vi "Validate TCP.vi"(8 "error in (no error)":errorcluster, 10 "User TCP Configuration":T1, 11 "LINX Resource":T2={"IO"=enum."Remote", "Interface"=enum."Serial", "LINX Device Config"={"Interface"=enum."Serial", "COM Port"="COM13", "TCP Configuration"={"IP Address"="", "Port"=0}, "Device Family"=1, "Device ID"=1, "Device Name"="myRIO-1900", "TCP Ref"=refnum, "Channels"={"DI"=[0, 1, 2, 3, 4, 5, 6, 7, 8, 9, 10, 11, 12, 13, 14, 15, 16, 17, 18, 19, 20, 21, 22, 23, 24, 25, 26, 27, 28, 29, 30, 31, 32, 33, 34, 35, 36, 37, 38, 39, 40, 41, 42, 43, 44, 45, 46], "DO"=[0, 1, 2, 3, 4, 5, 6, 7, 8, 9, 10, 11, 12, 13, 14, 15, 16, 17, 18, 19, 20, 21, 22, 23, 24, 25, 26, 27, 28, 29, 30, 31, 32, 33, 34, 35, 36, 37, 38, 39, 40, 41, 42, 43, 44, 45, 46], "AI"=[0, 1, 2, 3, 4, 5, 6, 7, 8, 9, 10, 11], "AO"=[], "PWM"=[3, 5, 6, 9, 10], "QE"=[], "UART"=[0, 1], "I2C 2"=[0], "SPI"=[0], "CAN"=[], "Servo"=[], "AI Ref (V)"=0.0, "AI Resolution (Bits)"=0, "AO Ref (V)"=0.0, "AO Resolution (Bits)"=0}}}) -> (0 "error out":errorcluster, 1 "WiFi status":u8, 2 "Board TCP Configuration":T1, 3 "LINX Resource Out":T2={"IO"=enum."Remote", "Interface"=enum."Serial", "LINX Device Config"={"Interface"=enum."Serial", "COM Port"="COM13", "TCP Configuration"={"IP Address"="", "Port"=0}, "Device Family"=1, "Device ID"=1, "Device Name"="myRIO-1900", "TCP Ref"=refnum, "Channels"={"DI"=[0, 1, 2, 3, 4, 5, 6, 7, 8, 9, 10, 11, 12, 13, 14, 15, 16, 17, 18, 19, 20, 21, 22, 23, 24, 25, 26, 27, 28, 29, 30, 31, 32, 33, 34, 35, 36, 37, 38, 39, 40, 41, 42, 43, 44, 45, 46], "DO"=[0, 1, 2, 3, 4, 5, 6, 7, 8, 9, 10, 11, 12, 13, 14, 15, 16, 17, 18, 19, 20, 21, 22, 23, 24, 25, 26, 27, 28, 29, 30, 31, 32, 33, 34, 35, 36, 37, 38, 39, 40, 41, 42, 43, 44, 45, 46], "AI"=[0, 1, 2, 3, 4, 5, 6, 7, 8, 9, 10, 11], "AO"=[], "PWM"=[3, 5, 6, 9, 10], "QE"=[], "UART"=[0, 1], "I2C 2"=[0], "SPI"=[0], "CAN"=[], "Servo"=[], "AI Ref (V)"=0.0, "AI Resolution (Bits)"=0, "AO Ref (V)"=0.0, "AO Resolution (Bits)"=0}}})   [LabVIEW 2019, in "LINXx.lvlib"]
doc: "Throw warning if IP/port do not match"
uses:
  LINXx.lvlib
  <vilib>/MakerHub/LINX/Private/Device/Type Defs/TCP Config.ctl
  <vilib>/MakerHub/LINX/Private/Type Defs/LINX Ref.ctl
  <vilib>/MakerHub/LINX/Private/Type Defs/Platform.ctl
  <vilib>/MakerHub/LINX/Private/Type Defs/Interface.ctl
  <vilib>/MakerHub/LINX/Private/Device/Type Defs/LINX Device Config.ctl
  <vilib>/MakerHub/LINX/Private/Device/Type Defs/Channels.ctl
  <vilib>/Utility/error.llb/Error Cluster From Error Code.vi
  <vilib>/ErrorRing/Error Ring.xnode
  <vilib>/MakerHub/LINX/Private/Device/Device.lvlib
  <vilib>/MakerHub/LINX/LMH-LINX.lvlib
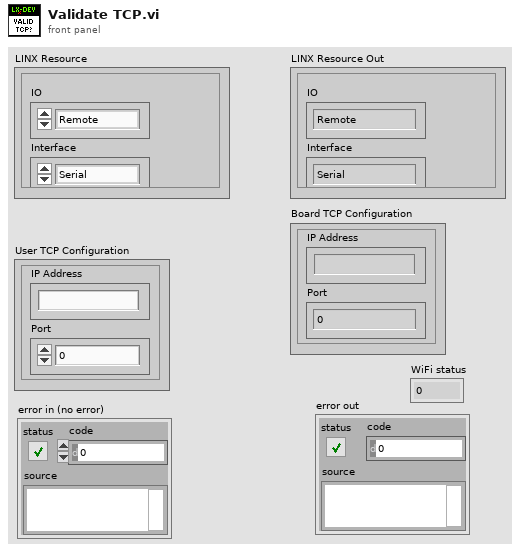
[diagram p1: front panel]
types:
  T1 = typedef "LMH-LINX.lvlib/Device.lvlib/TCP Config.ctl" = cluster{"IP Address":string, "Port":u16}
  T2 = typedef "LMH-LINX.lvlib/LINX Ref.ctl" = cluster{"IO":T3, "Interface":T4, "LINX Device Config":T5}
  T3 = typedef "LMH-LINX.lvlib/Platform.ctl" = enum16{"Remote", "Local"}
  T4 = typedef "LMH-LINX.lvlib/Interface.ctl" = enum16{"Serial", "TCP"}
  T5 = typedef "LMH-LINX.lvlib/Device.lvlib/LINX Device Config.ctl" = cluster{"Interface":T4, "COM Port":refnum<visa-resource-name>, "TCP Configuration":T1, "Device Family":u8, "Device ID":u8, "Device Name":string, "TCP Ref":refnum<k5>, "Channels":T6}
  T6 = typedef "LMH-LINX.lvlib/Channels.ctl" = cluster{"DI":u8[], "DO":u8[], "AI":u8[], "AO":u8[], "PWM":u8[], "QE":u8[], "UART":u8[], "I2C 2":u8[], "SPI":u8[], "CAN":u8[], "Servo":u8[], "AI Ref (V)":dbl, "AI Resolution (Bits)":u8, "AO Ref (V)":dbl, "AO Resolution (Bits)":u8}
  T7 = typedef "LMH-LINX.lvlib/Device.lvlib/Wifi Config.ctl" = cluster{"SSID":string, "IP Address":string, "Port":u16, "WIFI Security Type":T8, "Password":string}
  T8 = typedef "LMH-LINX.lvlib/WIFI Security Type.ctl" = enum8{"None", "WPA2 Password", "WPA2 Key", "WEP40", "WEP104"}
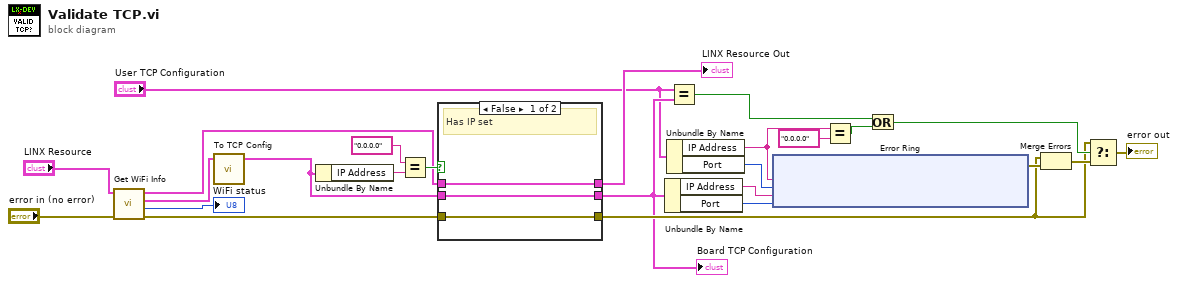
[diagram p0: block diagram]
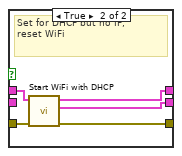
[diagram p2: hidden frame]
diagram:
  n1 = call "Get WiFi Info.vi"("Error In"="error in (no error)", "LINX Resource"="LINX Resource") -> ("Error Out"=w10:errorcluster, "WiFi status"=→"WiFi status":u8, "WiFi Info"=w17:T7, "LINX Resource Out"=w12:T2)  [unwired: 6 in]
  n2 = call "To TCP Config.vi"("Wifi Configuration"=w17) -> ("TCP Configuration"=w9:T1)  [unwired: 4 in]
  n3 = Unbundle By Name(w9) -> ("IP Address"=w14:string)
  n4 = Equal?(x="0.0.0.0" ("y"), y=w14) -> (x = y?=w13:bool)
  n5 = case shown="False" w13 {
    tunnel: w12 -> [w26 w33]
    tunnel: [w26 w32] -> w11
    tunnel: [w27 w31] -> w8
    tunnel: w10 -> [w27 w30]
    tunnel: [w28 w29] -> w3
    tunnel: w9 -> [w28 _]
    frame False {
      # "Has IP set"
    }
    frame True {
      # "Set for DHCP but no IP;\nreset WiFi"
      n6 = call "Start WiFi with DHCP.vi"("Error In"=w30, "LINX Resource"=w33) -> ("error out"=w31:errorcluster, "TCP Configuration Out"=w29:T1, "LINX Resource Out"=w32:T2)  [unwired: 7 in]
    }
  }
  "LINX Resource Out" <- w11
  "Board TCP Configuration" <- w3
  n7 = Unbundle By Name(w3) -> ("IP Address"=w5:string, "Port"=w4:u16)
  n8 = Unbundle By Name("User TCP Configuration") -> ("IP Address"=w1:string, "Port"=w6:u16)
  n9 = Equal?(x="User TCP Configuration", y=w3) -> (x = y?=w22:bool)
  n10 = xnode "Error Ring"("parameter 0"=w1, "parameter 1"=w6, "parameter 2"=w5, "parameter 3"=w4) -> ("error out"=w20:errorcluster)
  n11 = Equal?(x=w1, y="0.0.0.0") -> (x = y?=w25:bool)
  n12 = Or(x=w22, y=w25) -> (x .or. y?=w24:bool)
  n13 = Merge Errors(w8, w20) -> (w21:errorcluster)
  n14 = Select(t=w8, s=w24, f=w21) -> (s? t:f=→"error out":errorcluster)
